vi "set sim log.vi"(8 "error in (no error)":errorcluster, 11 "log":string) -> (0 "error out":errorcluster)   [LabVIEW 2019, in "libSimulationControl.lvlib"]
doc: "void set_sim_log(const char* log);"
uses:
  libSimulationControl.lvlib
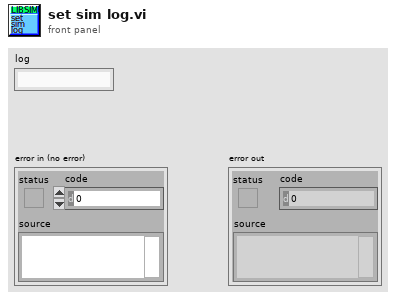
[diagram p1: front panel]
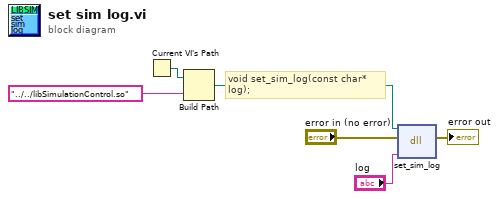
[diagram p0: block diagram]
diagram:
  # "void set_sim_log(const char* log);"
  n1 = Current VI's Path() -> (path=w3:path)
  n2 = Build Path(base path=w3, name or relative path="../../libSimulationControl.so") -> (appended path=w1:path)
  n3 = dll-call lib="home/paul/Schreibtisch/Biogas_plant_setup/LabView/lib/libSimulationControl/libSimulationControl.*" fn="set_sim_log"(path in=w1, error in="error in (no error)", "log"="log") -> (error out=→"error out":errorcluster)  [unwired: 3 in, 1 out]
